vi "Add Element.vi"(6 "Meta Data":T1[](array[typedef]), 8 "error in (no error)":errorcluster, 9 "Value":string, 10 "Hierarchy":string[](array[string]), 11 "Config Manager in":refnum<class "Config Manager.lvclass">) -> (0 "error out":errorcluster, 3 "Config Manager out":refnum<class "Config Manager.lvclass">)   [LabVIEW 2020]
uses:
  Config Manager.lvclass
  Config Element/Config Element.lvclass
  Meta Data.ctl
  CDM-Config.lvlib
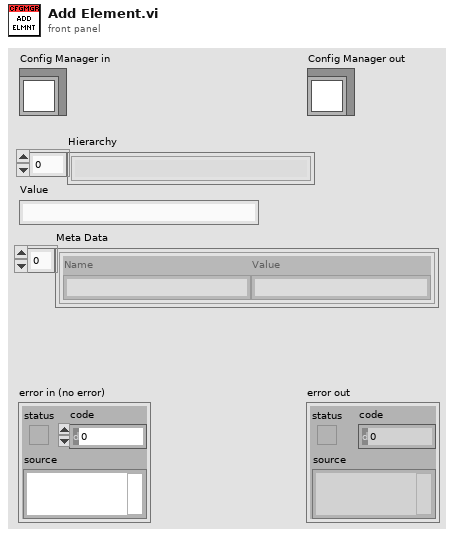
[diagram p1: front panel]
types:
  T1 = typedef "CDM-Config.lvlib/Meta Data.ctl" = cluster{"Name":string, "Value":string}
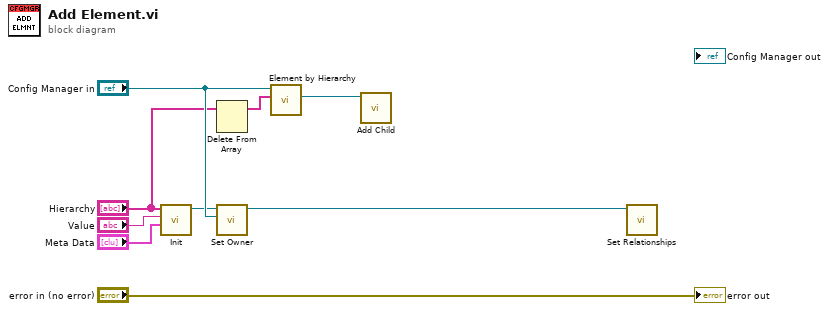
[diagram p0: block diagram]
diagram:
  n1 = call "Init.vi"("Meta Data"="Meta Data", "Value"="Value", "Hierarchy"="Hierarchy") -> ("Config Element out"=w6:refnum<class "Config Element.lvclass">)  [unwired: 7 in, 1 out]
  n2 = Delete From Array(array="Hierarchy") -> (array with subset deleted=w8:string[])  [unwired: 2 in, 1 out]
  n3 = call "Set Owner.vi"("Owner"="Config Manager in", "Config Element in"=w6) -> ("Config Element out"=w2:refnum<class "Config Element.lvclass">)  [unwired: 8 in, 1 out]
  n4 = call "Element by Hierarchy.vi"("Hierarchy"=w8, "Config Manager in"="Config Manager in") -> ("Config Element"=w1:refnum<class "Config Element.lvclass">)  [unwired: 7 in, 2 out]
  n5 = call "Add Child.vi"("Config Element in"=w1) -> ()  [unwired: 9 in, 2 out]
  n6 = call "Set Relationships.vi"("Config Element in"=w2) -> ()  [unwired: 9 in, 2 out]
  "error out" <- "error in (no error)"
